vi "create.noManifest_scale_factor.vi"(9 "scaleFactor":dbl=1.0, 10 "startingTimestamp":timestamp format="%<%x %.3X>T") -> (3 "Timestamp Manifest":refnum<class "noManifest.lvclass">)   [LabVIEW 2020, in "nominal types.lvlib" / "timestampManifest.lvlib"]
uses:
  timestampManifest.lvlib
  noManifest/noManifest.lvclass
  scaleFactor/scaleFactor.lvclass
  C:/code/labview-client/lv_src/nominal types/timestampManifest/scaleParameter/scaleParameter.lvclass
  scaleFactor/scaleFactor.lvclass/scaleFactor.ctl
  noManifest/noManifest.lvclass/noManifest.ctl
  scaleFactor/scaleFactor.set.vi
  noManifest/startingTimestamp.set.vi
  noManifest/scaleParameter.set.vi
  04c50cf6-0dc9-46a9-a5af-d1f05d95fae1.vi
  C:/code/labview-client/lv_src/Nominal Client/datasources/payload/payload.lvclass
  C:/code/labview-client/lv_src/nominal types/timestampManifest/scaleFactor/scaleFactor.lvclass
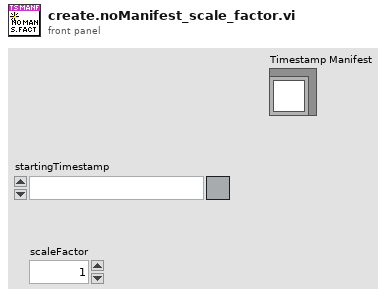
[diagram p1: front panel]
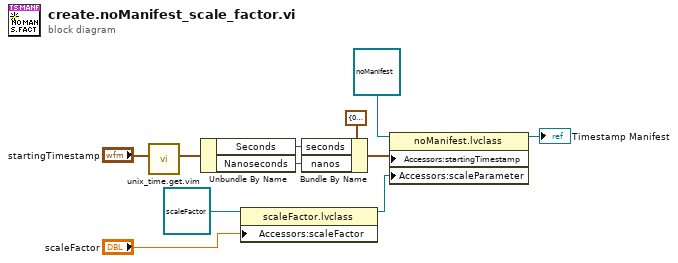
[diagram p0: block diagram]
diagram:
  n1 = call "unix_time.get.vim"("Time Stamp (empty: now) [single or array]"="startingTimestamp") -> ("UNIX Timestamp"=w3:cluster{"Seconds":i64, "Nanoseconds":i64})  [unwired: 10 in]
  n2 = Unbundle By Name(w3) -> ("Seconds"=w2:i64, "Nanoseconds"=w1:i64)
  n3 = property class="scaleFactor.lvclass"(reference=refnum<class "scaleFactor.lvclass"> refnum ("nominal types.lvlib:timestampManifest.lvlib:scaleFactor.lvclass"), "Accessors:scaleFactor"="scaleFactor") -> (reference out=w8:refnum<class "scaleFactor.lvclass">)  [unwired: 1 in, 1 out]
  n4 = Bundle By Name(cluster=cluster{"seconds":i64, "nanos":i64, "picos":i64} {"seconds"=0, "nanos"=0, "picos"=0} ("startingTimestamp"), "seconds"=w2, "nanos"=w1) -> (w4:cluster{"seconds":i64, "nanos":i64, "picos":i64})
  n5 = property class="noManifest.lvclass"(reference=refnum<class "noManifest.lvclass"> refnum ("nominal types.lvlib:timestampManifest.lvlib:noManifest.lvclass"), "Accessors:startingTimestamp"=w4, "Accessors:scaleParameter"=w8) -> (reference out=→"Timestamp Manifest":refnum<class "noManifest.lvclass">)  [unwired: 1 in, 1 out]
